vi "Read Temperature.vi"(8 "error in (no error)":errorcluster, 11 "CCDCamera in":refnum<class "CCDCamera.lvclass">) -> (0 "error out":errorcluster, 2 "Temperature":i32=20 min=0 max=0, 3 "CCDCamera out":refnum<class "CCDCamera.lvclass">)   [LabVIEW 2018, in "CCDCamera.lvclass"]
uses:
  CCDCamera.lvclass
  CCDCamera.lvclass/CCDCamera.ctl
  Cooler/Cooler.lvclass
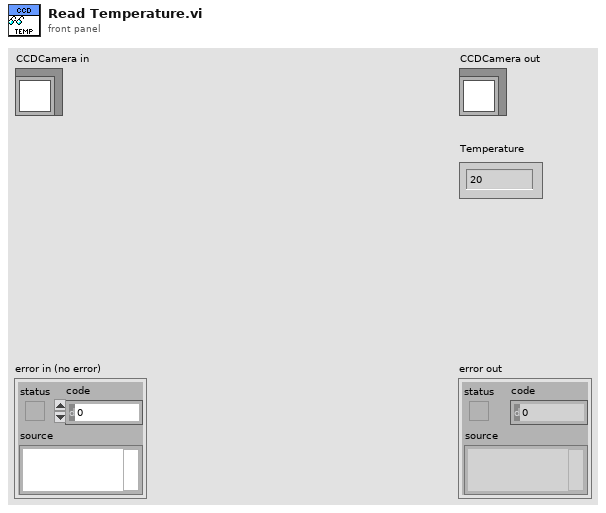
[diagram p1: front panel]
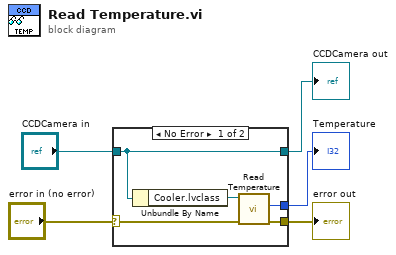
[diagram p0: block diagram]
diagram:
  n1 = case shown="No Error" "error in (no error)" {
    selector: "error in (no error)" -> [w8 w11]
    tunnel: [w9 w11] -> w4
    tunnel: [w10 w12] -> w2
    tunnel: "CCDCamera in" -> [w10 w12]
    tunnel: [w6 _] -> w1
    frame No Error {
      n2 = Unbundle By Name(w10) -> ("Cooler.lvclass"=w7:refnum<class "Cooler.lvclass">)
      n3 = call-dynamic "Read Temperature.vi"("error in (no error)"=w8, "Cooler in"=w7) -> ("error out"=w9:errorcluster, "Temperature"=w6:i32)  [unwired: 7 in, 1 out]
    }
    frame Error {
    }
  }
  "error out" <- w4
  "CCDCamera out" <- w2
  "Temperature" <- w1
